vi "Refresh Listbox.vi"(11 "ListboxBusMonitorPanel in":refnum<class "ListboxBusMonitorPanel.lvclass">) -> (3 "ListboxBusMonitorPanel out":refnum<class "ListboxBusMonitorPanel.lvclass">)   [LabVIEW 2017, in "ListboxBusMonitor.lvlib" / "ListboxBusMonitorPanel.lvclass"]
uses:
  <vilib>/gpm_packages/@cs/BusMonitor/ListboxBusMonitor/ListboxBusMonitorPanel/ListboxBusMonitorPanel.lvclass
  <vilib>/gpm_packages/@cs/BusMonitor/ListboxBusMonitor/ListboxBusMonitorPanel/ListboxBusMonitorPanel.lvclass/ListboxBusMonitorPanel.ctl
panel:
  in  "Cluster":T1
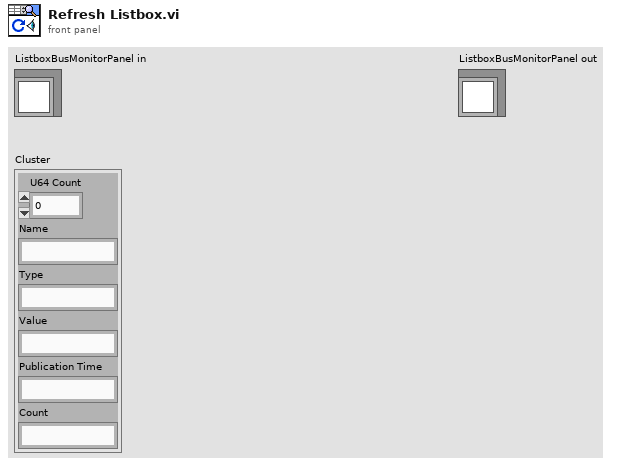
[diagram p1: front panel]
types:
  T1 = cluster{"U64 Count":u64, "Name":string, "Type":string, "Value":string, "Publication Time":string, "Count":string}
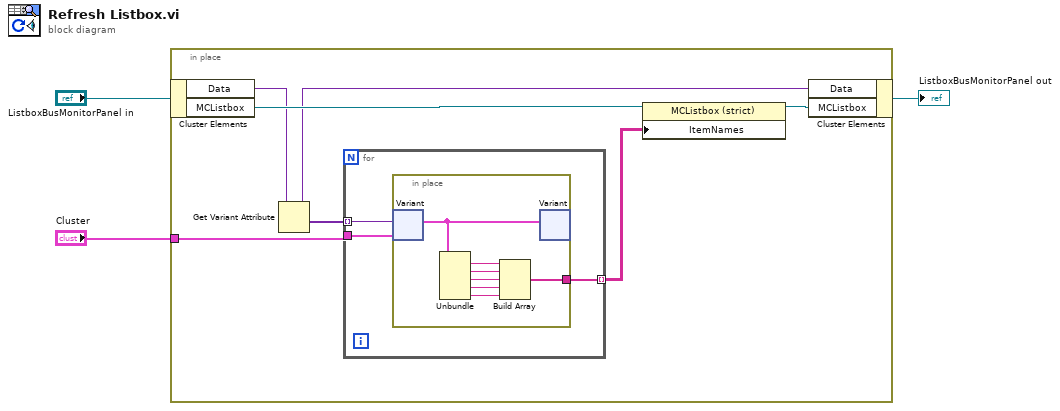
[diagram p0: block diagram]
diagram:
  n1 = in-place {
    in-place-border: "Cluster" -> [w4]
    n2 = in-place-cluster #1("ListboxBusMonitorPanel in") -> ("Data"=w8:variant, "MCListbox"=w10:refnum<vi>)
    n3 = Get Variant Attribute(Variant=w8) -> (duplicate Variant=w7:variant, values=w6:variant[])  [unwired: 3 in, 2 out]
    n4 = for {
      tunnel: w6 -> [w13] mode=indexing
      tunnel: w4 -> [w12]
      tunnel: [w11] -> w5 mode=indexing
      n5 = in-place {
        in-place-border: [w19] -> w11
        n6 = in-place-variant #2(w13, w12) -> (w20:T1)  [unwired: 1 out]
        n7 = Unbundle(w20) -> ("Name"=w18:string, "Type"=w17:string, "Value"=w16:string, "Publication Time"=w15:string, "Count"=w14:string)  [unwired: 1 out]
        n8 = Build Array(w18, w17, w16, w15, w14) -> (w19:string[])
        n9 = in-place-variant #2(w20) -> ()  [unwired: 2 out]
      }
    }
    n10 = property class="MCListbox (strict)"(reference=w10, "ItemNames"=w5) -> (reference out=w9:refnum<vi>)  [unwired: 1 in, 1 out]
    n11 = in-place-cluster #1("Data"=w7, "MCListbox"=w9) -> (→"ListboxBusMonitorPanel out":refnum<class "ListboxBusMonitorPanel.lvclass">)
  }
